vi "labview part b.vi"() -> ()   [LabVIEW 2011]
panel:
  in  "stop":bool
  out "Waveform Chart":dbl[](graph)
  out "Thermometer":dbl(slide) scale=0.0..100.0
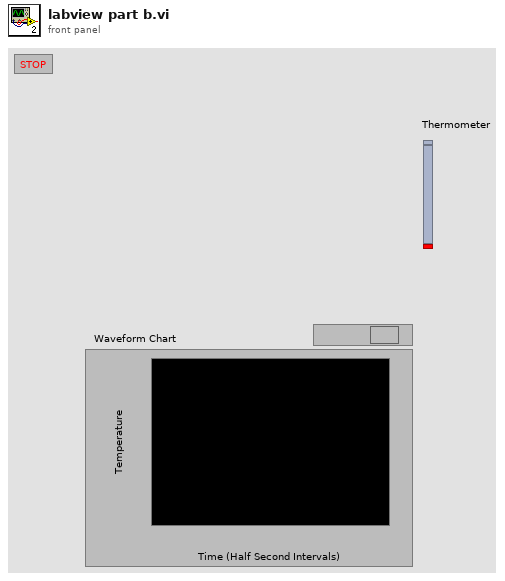
[diagram p1: front panel]
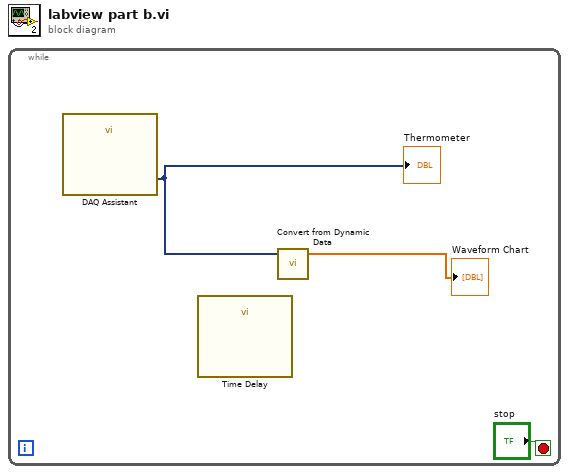
[diagram p0: block diagram]
diagram:
  n1 = while {
    stop <- "stop" stop-if-true
    n2 = call "DAQ Assistant"() -> ("data"=w2:dynamicdata)  [unwired: 17 in, 2 out]
    "Thermometer" <- w2
    n3 = call "Time Delay"() -> ()  [unwired: 11 in, 1 out]
    n4 = call "Convert from Dynamic Data"("Dynamic Data Type"=w2) -> ("Array"=→"Waveform Chart":dbl[])  [unwired: 3 in]
  }
